vi "Alarm.vi"(9 "error in (no error)":errorcluster, 10 "Alarm Time (s)":dbl) -> (1 "error out":errorcluster)   [LabVIEW 2010]
doc: "This VI serves as an alarm and waits the input time (seconds) before allowing program operation to continue.\n\nInputs:\nAlarm Time (s) - amount of time to wait before continuing\nerror in - error input cluster\n\nOutputs:\nerror out - error output cluster"
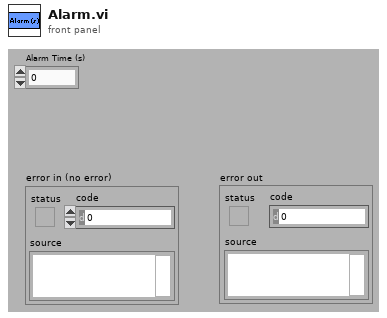
[diagram p1: front panel]
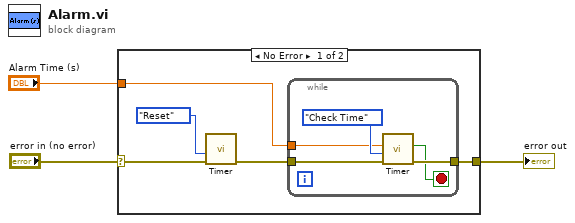
[diagram p0: block diagram]
diagram:
  n1 = case shown="No Error" "error in (no error)" {
    selector: "error in (no error)" -> [w5 w14]
    tunnel: [w6 w14] -> w2
    tunnel: "Alarm Time (s)" -> [w4 _]
    frame No Error {
      n2 = call <userlib>:"Timer.vi"("error in (no error)"=w5, "Command"=enum16{"Reset", "Get Time", "Check Time"}."Reset") -> ("error out"=w7:errorcluster)  [unwired: 7 in, 2 out]
      n3 = while {
        tunnel: w7 -> [w12]
        tunnel: [w11] -> w6
        tunnel: w4 -> [w10]
        stop <- w9 stop-if-true
        n4 = call <userlib>:"Timer.vi"("error in (no error)"=w12, "Command"=enum16{"Reset", "Get Time", "Check Time"}."Check Time", "Wait Time (s)"=w10) -> ("error out"=w11:errorcluster, "Time Expired?"=w9:bool)  [unwired: 6 in, 1 out]
      }
    }
    frame Error {
    }
  }
  "error out" <- w2
